vi "SaveAs Document.vi"(8 "error in (no error)":errorcluster, 10 "Document Path":path, 11 "Document API in":refnum<class "Document API.lvclass">) -> (0 "error out":errorcluster, 3 "Document API out":refnum<class "Document API.lvclass">)   [LabVIEW 2017, in "Document API.lvlib" / "Document API.lvclass"]
doc: "Saves the <b>Document</b> to the given <b>Document Path</b>.\n\nNotes:\n - If <b>Document Path</b> is empty (default) or is <Not A Path> or is a directory, the VI displays a dialog box from which the user can select a file. Error 43 occurs if you cancel the dialog box. \n - If the <b>Document Path</b> already contains a docuement with the same name then that file is overwritten without warning."
uses:
  Document API.lvclass
  Document API.lvclass/Document API.ctl
  NPOI_Document/npoiDocument/npoiDocument.lvclass
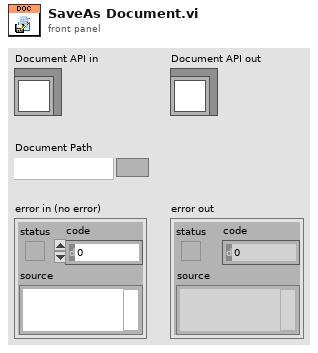
[diagram p1: front panel]
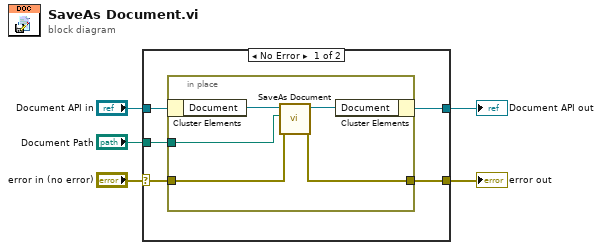
[diagram p0: block diagram]
diagram:
  n1 = case shown="No Error" "error in (no error)" {
    selector: "error in (no error)" -> [w8 w17]
    tunnel: [w7 w17] -> w4
    tunnel: [w10 w16] -> w2
    tunnel: "Document API in" -> [w9 w16]
    tunnel: "Document Path" -> [w6 _]
    frame No Error {
      n2 = in-place {
        in-place-border: w8 -> [w13]
        in-place-border: [w12] -> w7
        in-place-border: w6 -> [w11]
        n3 = in-place-cluster #1(w9) -> ("Document"=w15:refnum<class "npoiDocument.lvclass">)
        n4 = call "SaveAs Document.vi"("error in (no error)"=w13, "Document Path"=w11, "Document in"=w15) -> ("error out"=w12:errorcluster, "Document out"=w14:refnum<class "npoiDocument.lvclass">)  [unwired: 7 in]
        n5 = in-place-cluster #1("Document"=w14) -> (w10:refnum<class "Document API.lvclass">)
      }
    }
    frame Error {
    }
  }
  "error out" <- w4
  "Document API out" <- w2
